vi "reportHPServerID.vi"(0 "ILCCommunication in":refnum<class "ILCCommunication.lvclass">, 5 "HPIndex":i32, 7 "WaitForTrigger":bool, 9 "TriggerIRQ":bool, 11 "error in (no error)":errorcluster) -> (4 "ILCCommunication out":refnum<class "ILCCommunication.lvclass">, 15 "error out":errorcluster)   [LabVIEW 2016, in "ILCCommunication.lvclass"]
uses:
  ILCCommunication.lvclass
  ILCCommunication.lvclass/ILCCommunication.ctl
  Common_RT_HPILC/HPILC/HPILC.lvclass
  D:/Code/ts_M1M3Support/Common_RT_ILC/ILC/ILC.lvclass
  Common_RT_Modbus/IModbus/IModbus.lvclass
  Common_RT_ILC/ILC/ILC.lvclass
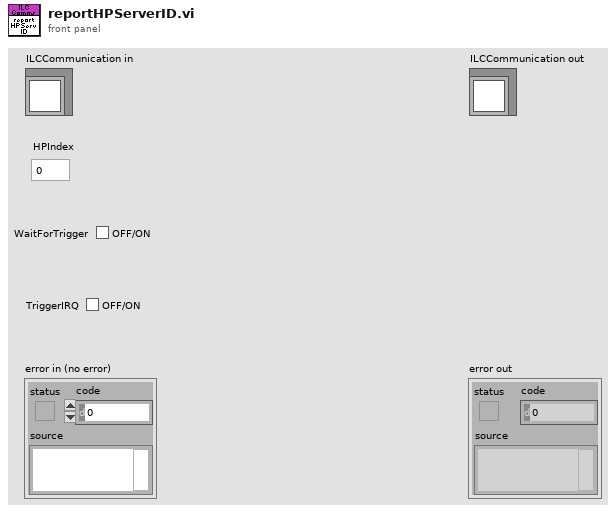
[diagram p1: front panel]
types:
  T1 = typedef "RTModbus.lvlib/TxFrame.ctl" = cluster{"Data":u8[], "WaitForTrigger":bool, "WaitForRx":u16, "TriggerIRQ":bool, "DelayMicroseconds":u16, "DelayMilliseconds":u16, "Timestamp":bool}
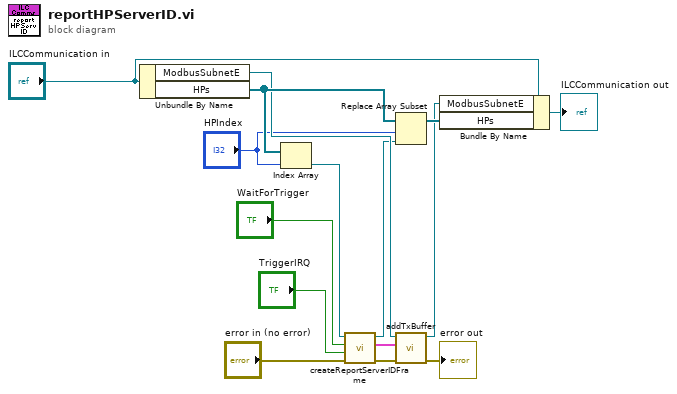
[diagram p0: block diagram]
diagram:
  n1 = Unbundle By Name("ILCCommunication in") -> ("ModbusSubnetE"=w12:refnum<class "IModbus.lvclass">, "HPs"=w13:refnum<class "HPILC.lvclass">[])
  n2 = Index Array(array=w13, index="HPIndex") -> (element=w6:refnum<class "HPILC.lvclass">)
  n3 = call "createReportServerIDFrame.vi"("error in (no error)"="error in (no error)", "TriggerIRQ"="TriggerIRQ", "WaitForTrigger"="WaitForTrigger", "ILC in"=w6) -> ("error out"=w3:errorcluster, "TxFrame"=w5:T1, "ILC out"=w4:refnum<class "HPILC.lvclass">)  [unwired: 5 in]
  n4 = Replace Array Subset(array=w13, new element=w4, index="HPIndex") -> (w15:refnum<class "HPILC.lvclass">[])
  n5 = call-dynamic "addTxBuffer.vi"("error in (no error)"=w3, "TxFrame"=w5, "IModbus in"=w12) -> ("error out"=→"error out":errorcluster, "IModbus out"=w14:refnum<class "IModbus.lvclass">)  [unwired: 7 in]
  n6 = Bundle By Name(cluster="ILCCommunication in", "ModbusSubnetE"=w14, "HPs"=w15) -> (→"ILCCommunication out":refnum<class "ILCCommunication.lvclass">)
